vi "capacitance navigation xy.vi"() -> ()   [LabVIEW 2010]
uses:
  <userlib>/Nanonis Prog Interface V5/Nanonis Prog Interface.lvlib
panel:
  out "Capacitance Z":cluster{"index":i32, sgl}[](graph)
  out "Avg index 3":i32
  out "Avg index 2":i32
  in  "pause":bool
  in  "Delete First Entry":bool
  in  "Time between averages (ms)":u32
  out "Avg index":i32
  in  "Averages":i32=50
  in  "milliseconds to wait":u32=1000
  in  "stop":bool
  in  "?":bool
  in  "Max Steps":u16=500
  in  "Direction":enum16{"X +", "X -", "Y +", "Y -", "Z +", "Z -"}(ring)
  out "Capacitance Y":cluster{"index":i32, sgl}[](graph)
  in  "Number of Steps":u16=50
  out "Capacitance X":cluster{"index":i32, sgl}[](graph)
  in  "Frequency (Hz)":sgl=261.0
  in  "Amplitude (V)":sgl=350.0
  # "Max Steps On"
  # "Max Steps Off"
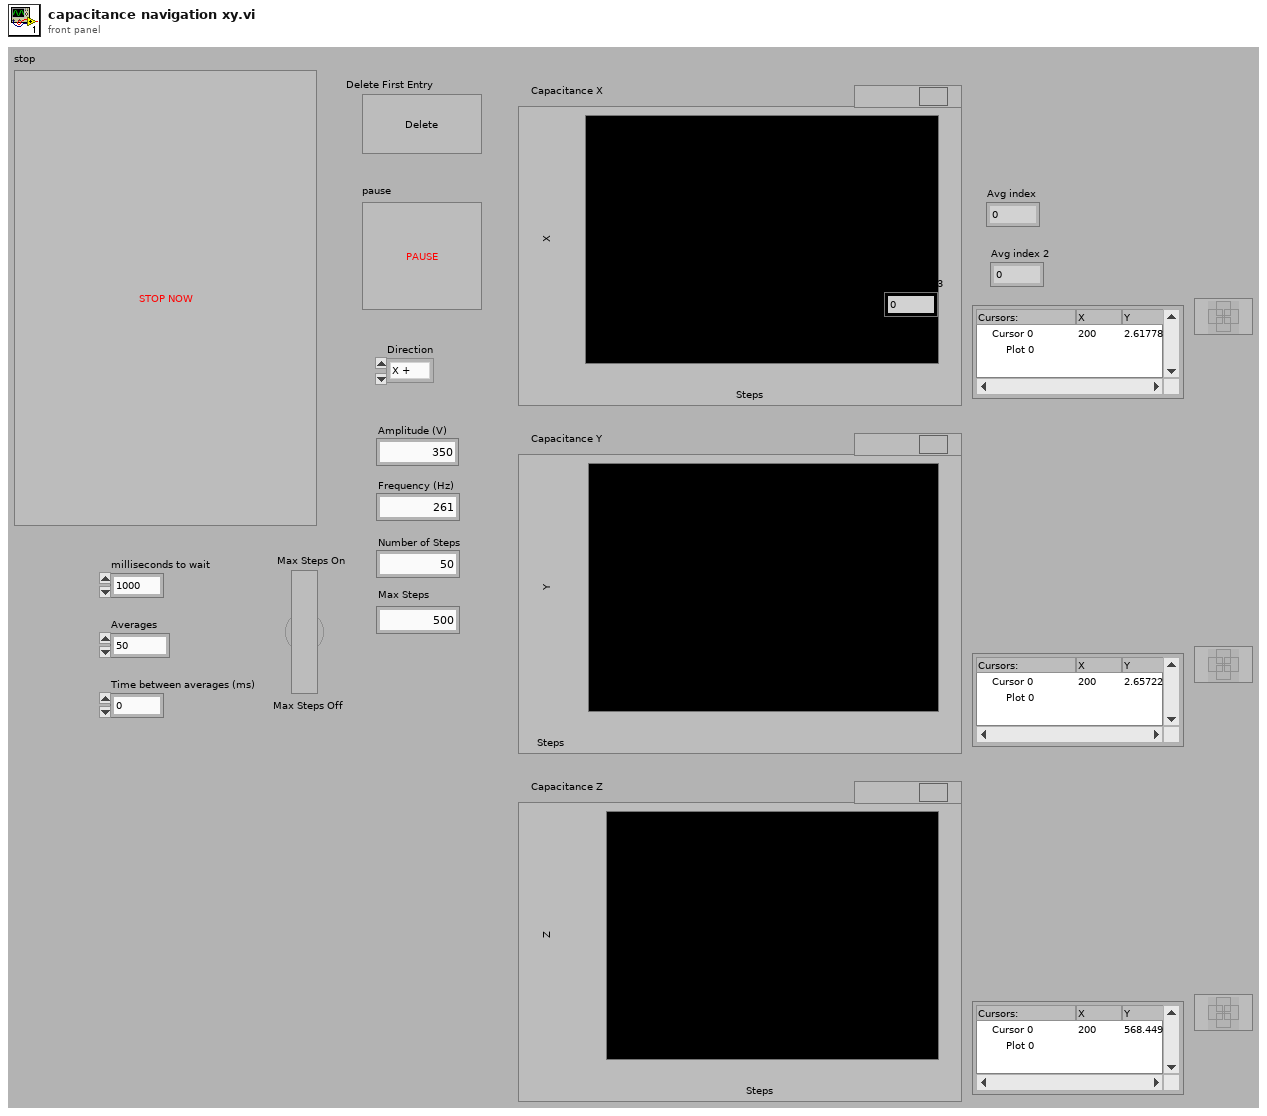
[diagram p1: front panel]
types:
  T1 = enum8{"Group 1", "Group 2", "Group 3", "Group 4", "Group 5", "Group 6"}
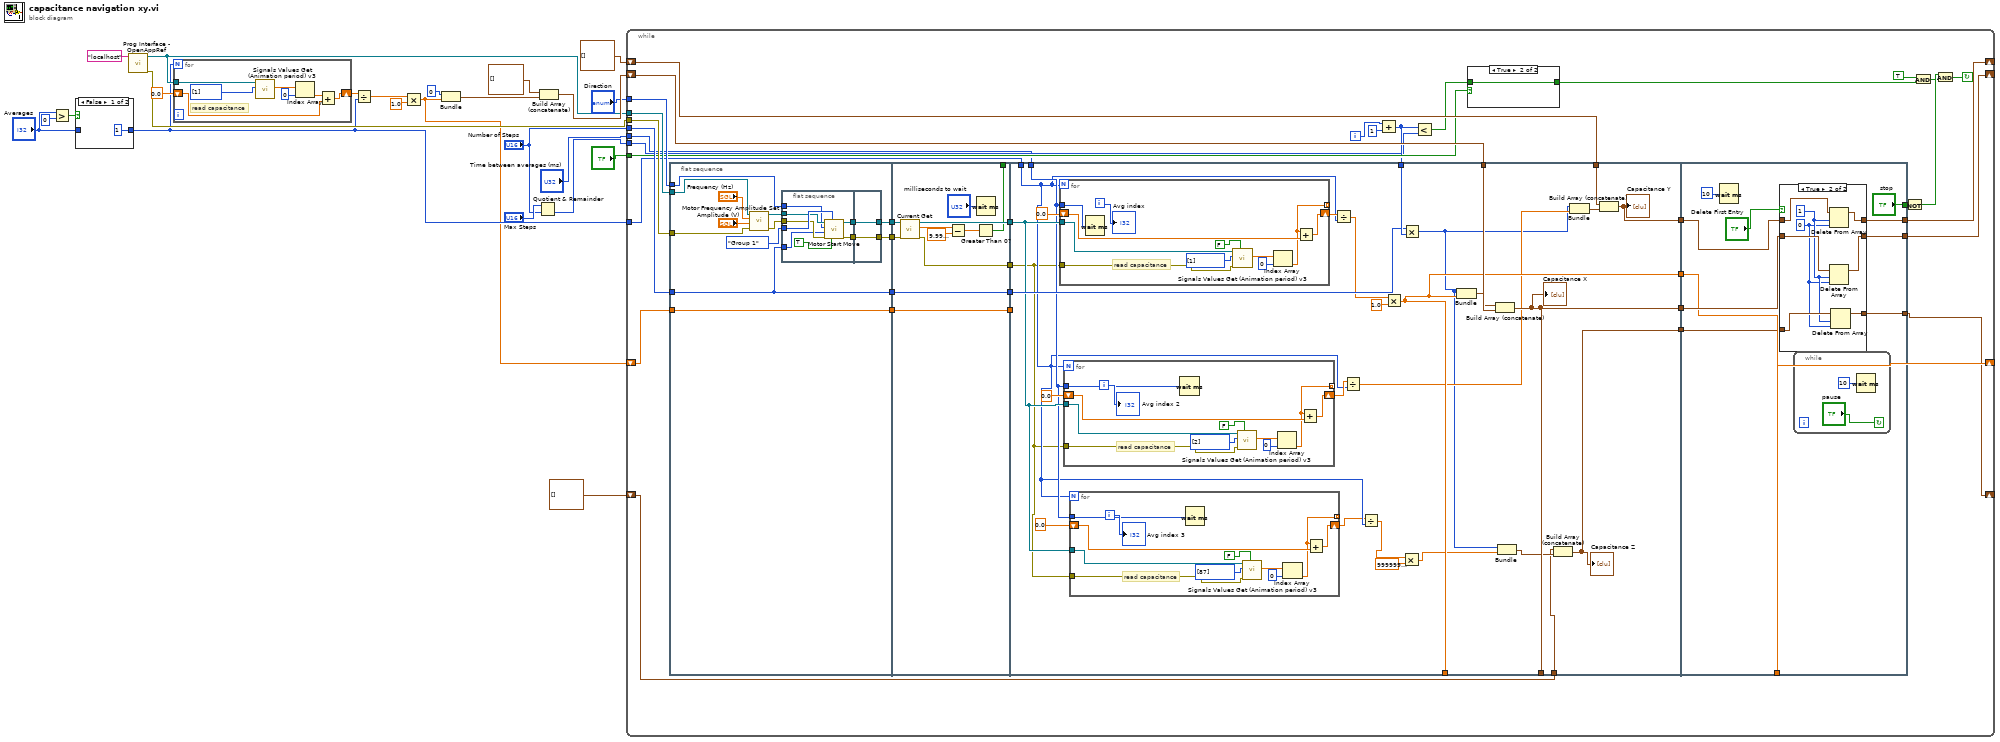
[diagram p0: block diagram]
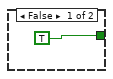
[diagram p3: hidden frame]
diagram:
  n1 = Greater?(x="Averages", y=0) -> (0:w9:bool)
  n2 = case shown="False" w9 {
    tunnel: "Averages" -> [_ w26]
    tunnel: [1 ("Averages") w26] -> w4
    frame False {
    }
    frame True {
    }
  }
  n3 = call <userlib>:"Prog Interface - OpenAppRef.vi"("Machine name (local machine IP)"="localhost" ("machine name (localhost)")) -> ("Error out"=w18:errorcluster, "Application reference"=w17:refnum<vi>)  [unwired: 5 in]
  n4 = for {
    N: w4 -> [_]
    tunnel: w17 -> [w30]
    shift-right: [w27] -> w5
    shift-left: sgl 0.0 ("Internal Ch Value") -> [w29]
    # "read capacitance"
    n5 = call <userlib>:"Signals Values Get (Animation period) v3.vi"("Signals indexes (0-127)"=i8[] [1], "Application ref in"=w30) -> ("Signals Values"=w31:sgl[])  [unwired: 6 in, 2 out]
    n6 = Index Array(array=w31, index=0) -> (element=w28:sgl)
    n7 = Add(x=w28, y=w29) -> (x+y=w27:sgl)
  }
  n8 = Divide(x=w5, y=w4) -> (x/y=w3:sgl)
  n9 = Multiply(x=w3, y=sgl 1.0) -> (x*y=w2:sgl)
  n10 = Bundle("index"=0, w2) -> (w21:cluster{"index":i32, sgl})  [unwired: 1 in]
  n11 = Quotient & Remainder(x="Max Steps", y="Number of Steps") -> (floor(x/y)=w12:u16)  [unwired: 1 out]
  n12 = Build Array (concatenate)(cluster{i32, sgl}[] [], w21) -> (w20:cluster{"index":i32, sgl}[])
  n13 = while {
    shift-right: [w42] -> _
    shift-left: w20 -> [w69]
    tunnel: w17 -> [w67]
    tunnel: w18 -> [w66]
    shift-right: [w60] -> _
    shift-left: cluster{i32, sgl}[] [] -> [w59]
    tunnel: "Direction" -> [w58]
    tunnel: "Number of Steps" -> [w57]
    tunnel: w12 -> [w50]
    tunnel: "?" -> [w56]
    tunnel: w4 -> [w45]
    tunnel: "Time between averages (ms)" -> [w44]
    shift-right: [w40] -> _
    shift-left: w2 -> [w39]
    shift-right: [w34] -> _
    shift-left: cluster{i32, sgl}[] [] -> [w36]
    i -> [w53]
    stop <- w47 continue-if-true
    n14 = flat-sequence {
      tunnel: [w76] -> w71
      tunnel: w67 -> [w79]
      tunnel: w66 -> [w82]
      tunnel: [w81] -> w65
      tunnel: [w80] -> w64
      tunnel: w58 -> [w75]
      tunnel: w57 -> [w76]
      tunnel: w39 -> [w74]
      tunnel: [w74] -> w38
      tunnel: w71 -> [w108]
      tunnel: [w108] -> w70
      tunnel: w65 -> [w107]
      tunnel: w64 -> [w106]
      tunnel: [w105] -> w63
      tunnel: [w104] -> w62
      tunnel: [w101] -> _
      tunnel: w38 -> [w98]
      tunnel: [w98] -> w37
      tunnel: [w126] -> _
      tunnel: w51 -> [w136]
      tunnel: w70 -> [w133]
      tunnel: w69 -> [w134]
      tunnel: [w125] -> _
      tunnel: w63 -> [w109]
      tunnel: w62 -> [w120]
      tunnel: [w130] -> w61
      tunnel: w59 -> [w131]
      tunnel: w45 -> [w116]
      tunnel: w44 -> [w119]
      tunnel: [w126] -> w43
      tunnel: [w125] -> w41
      tunnel: w37 -> [_]
      tunnel: w36 -> [w111]
      tunnel: [w110] -> w35
      tunnel: w61 -> [w178]
      tunnel: [w177] -> w60
      tunnel: ["stop"] -> w46
      tunnel: [w175] -> w42
      tunnel: w43 -> [w176]
      tunnel: w41 -> [w174]
      tunnel: [w174] -> w40
      tunnel: w35 -> [w172]
      tunnel: [w171] -> w34
      frame #0 {
        n15 = call <userlib>:"Motor Frequency Amplitude Set.vi"("Error in (no error)"=w82, "Amplitude (V) (NaN=no change)"="Amplitude (V)", "Frequency (Hz) (NaN=no change)"="Frequency (Hz)", "Application ref in"=w79) -> ("Error out"=w83:errorcluster, "Application ref out"=w84:refnum<vi>)  [unwired: 6 in]
        n16 = flat-sequence {
          tunnel: T1."Group 1" ("Group") -> [w94]
          tunnel: w84 -> [w93]
          tunnel: w83 -> [w92]
          tunnel: w76 -> [w91]
          tunnel: [w90] -> w78
          tunnel: [w89] -> w77
          tunnel: w75 -> [w88]
          tunnel: [w96] -> w80
          tunnel: [w97] -> w81
          tunnel: w78 -> [w97]
          tunnel: w77 -> [w96]
          frame #0 {
            n17 = call <userlib>:"Motor Start Move.vi"("Wait until finished? (F)"=TRUE, "Group"=w94, "Error in (no error)"=w92, "Number of steps"=w91, "Direction"=w88, "Application ref in"=w93) -> ("Error out"=w89:errorcluster, "Application ref out"=w90:refnum<vi>)  [unwired: 3 in]
          }
          frame #1 {
          }
        }
      }
      frame #1 {
        n18 = call <userlib>:"Current Get.vi"("Error in (no error)"=w106, "Application ref in"=w107) -> ("Error out"=w105:errorcluster, "Current (A)"=w103:sgl, "Application ref out"=w104:refnum<vi>)  [unwired: 5 in]
        n19 = Subtract(x=w103, y=sgl 1e-09) -> (x-y=w102:sgl)
        n20 = Greater Than 0?(x=w102) -> (x > 0?=w101:bool)
        n21 = Wait (ms)(milliseconds to wait="milliseconds to wait") -> ()  [unwired: 1 out]
      }
      frame #2 {
        n22 = for {
          N: w116 -> [_]
          tunnel: w109 -> [w167]
          tunnel: w120 -> [w166]
          shift-right: [w164] -> w128
          shift-left: sgl 0.0 ("y") -> [w165]
          tunnel: w119 -> [w162]
          tunnel: [w160] -> _ mode=indexing
          i -> [w163]
          # "read capacitance"
          n23 = Wait (ms)(milliseconds to wait=w162) -> ()  [unwired: 1 out]
          n24 = call <userlib>:"Signals Values Get (Animation period) v3.vi"("Wait for newest data (F=False)"=FALSE, "error in (no error)"=w167, "Signals indexes (0-127)"=i8[] [1], "Application ref in"=w166) -> ("Signals Values"=w168:sgl[])  [unwired: 4 in, 2 out]
          n25 = Index Array(array=w168, index=0) -> (element=w160:sgl)
          n26 = Add(x=w160, y=w165) -> (x+y=w164:sgl)
          "Avg index" <- w163
        }
        n27 = for {
          N: w116 -> [_]
          tunnel: w109 -> [w156]
          tunnel: w120 -> [w155]
          shift-right: [w153] -> w124
          shift-left: sgl 0.0 ("y") -> [w154]
          tunnel: w119 -> [w151]
          tunnel: [w149] -> _ mode=indexing
          i -> [w152]
          # "read capacitance"
          n28 = Wait (ms)(milliseconds to wait=w151) -> ()  [unwired: 1 out]
          n29 = call <userlib>:"Signals Values Get (Animation period) v3.vi"("Wait for newest data (F=False)"=FALSE, "error in (no error)"=w156, "Signals indexes (0-127)"=i8[] [2], "Application ref in"=w155) -> ("Signals Values"=w157:sgl[])  [unwired: 4 in, 2 out]
          n30 = Index Array(array=w157, index=0) -> (element=w149:sgl)
          n31 = Add(x=w149, y=w154) -> (x+y=w153:sgl)
          "Avg index 2" <- w152
        }
        n32 = for {
          N: w116 -> [_]
          tunnel: w109 -> [w138]
          tunnel: w120 -> [w145]
          shift-right: [w143] -> w112
          shift-left: sgl 0.0 ("y") -> [w144]
          tunnel: w119 -> [w141]
          tunnel: [w139] -> _ mode=indexing
          i -> [w142]
          # "read capacitance"
          n33 = Wait (ms)(milliseconds to wait=w141) -> ()  [unwired: 1 out]
          n34 = call <userlib>:"Signals Values Get (Animation period) v3.vi"("Wait for newest data (F=False)"=FALSE, "error in (no error)"=w138, "Signals indexes (0-127)"=i8[] [87], "Application ref in"=w145) -> ("Signals Values"=w146:sgl[])  [unwired: 4 in, 2 out]
          n35 = Index Array(array=w146, index=0) -> (element=w139:sgl)
          n36 = Add(x=w139, y=w144) -> (x+y=w143:sgl)
          "Avg index 3" <- w142
        }
        n37 = Divide(x=w128, y=w116) -> (x/y=w127:sgl)
        n38 = Divide(x=w124, y=w116) -> (x/y=w122:sgl)
        n39 = Divide(x=w112, y=w116) -> (x/y=w117:sgl)
        n40 = Multiply(x=w127, y=sgl 1.0) -> (x*y=w125:sgl)
        n41 = Multiply(x=w117, y=sgl 1000000000000.0) -> (x*y=w114:sgl)
        n42 = Multiply(x=w133, y=w136) -> (x*y=w115:i32)
        n43 = Bundle(w115, w125) -> (w135:cluster{i32, sgl})  [unwired: 1 in]
        n44 = Build Array (concatenate)(w134, w135) -> (w126:cluster{"index":i32, sgl}[])
        "Capacitance X" <- w126
        n45 = Bundle(w115, w114) -> (w113:cluster{i32, sgl})  [unwired: 1 in]
        n46 = Build Array (concatenate)(w111, w113) -> (w110:cluster{i32, sgl}[])
        "Capacitance Z" <- w110
        n47 = Bundle(w115, w122) -> (w132:cluster{i32, sgl})  [unwired: 1 in]
        n48 = Build Array (concatenate)(w131, w132) -> (w130:cluster{i32, sgl}[])
        "Capacitance Y" <- w130
      }
      frame #3 {
        n49 = Wait (ms)(milliseconds to wait=u32 10) -> ()  [unwired: 1 out]
        n50 = case shown="True" "Delete First Entry" {
          tunnel: w178 -> [w185 w193]
          tunnel: [w185 w192] -> w177
          tunnel: w176 -> [w184 w190]
          tunnel: [w184 w191] -> w175
          tunnel: w172 -> [w183 w189]
          tunnel: [w183 w188] -> w171
          frame False {
          }
          frame True {
            w187 = 1 ("length")
            w186 = 0 ("index")
            n51 = Delete From Array(array=w193, length=w187, index=w186) -> (array with subset deleted=w192:cluster{i32, sgl}[])  [unwired: 1 out]
            n52 = Delete From Array(array=w190, length=w187, index=w186) -> (array with subset deleted=w191:cluster{"index":i32, sgl}[])  [unwired: 1 out]
            n53 = Delete From Array(array=w189, length=w187, index=w186) -> (array with subset deleted=w188:cluster{i32, sgl}[])  [unwired: 1 out]
          }
        }
        n54 = while {
          stop <- "pause" continue-if-true
          n55 = Wait (ms)(milliseconds to wait=u32 10) -> ()  [unwired: 1 out]
        }
      }
    }
    n56 = Add(x=w53, y=u16 1) -> (x+y=w51:i32)
    n57 = Less?(x=w51, y=w50) -> (x < y?=w52:bool)
    n58 = case shown="True" w56 {
      tunnel: w52 -> [_ w73]
      tunnel: [TRUE w73] -> w54
      frame False {
      }
      frame True {
      }
    }
    n59 = Not(x=w46) -> (.not. x?=w49:bool)
    n60 = And(x=TRUE, y=w54) -> (x .and. y?=w48:bool)
    n61 = And(x=w49, y=w48) -> (x .and. y?=w47:bool)
  }
